vi "sheshen.vi"(3 "数组":cluster{"数值":dbl, "数值 2":dbl}[](array[cluster])) -> (1 "逻辑或":bool)   [LabVIEW 2009]
doc: "当蛇身大于等于5时判断蛇头是否和蛇身碰撞！若碰撞返回一个ture结束游戏，否则返回false游戏继续！"
uses:
  Global 3.vi
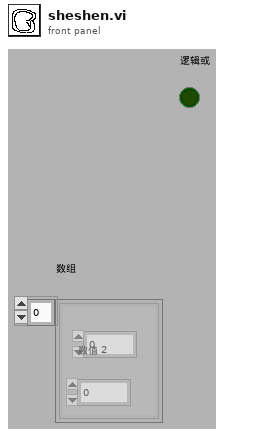
[diagram p1: front panel]
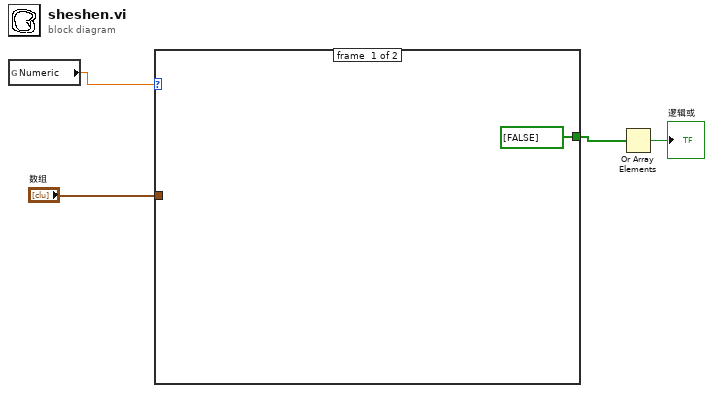
[diagram p0: block diagram]
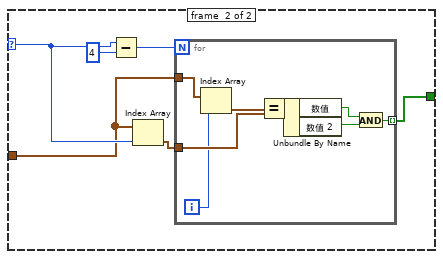
[diagram p2: hidden frame]
diagram:
  n1 = global read "Global 3.vi" "Numeric"() -> (w4:dbl)
  n2 = case shown="5, 默认" w4 {
    selector: w4 -> [_ w9]
    tunnel: "数组" -> [_ w6]
    tunnel: [bool[] [FALSE] w7] -> w2
    frame #0 {
    }
    frame #1 {
      n3 = Subtract(x=w9, y=4) -> (x-y=w10:i32)
      n4 = Index Array(array=w6, index=w9) -> (element=w8:cluster{"数值":dbl, "数值 2":dbl})
      n5 = for {
        N: w10 -> [_]
        tunnel: w6 -> [w19]
        tunnel: w8 -> [w17]
        tunnel: [w13] -> w7 mode=indexing
        i -> [w12]
        n6 = Index Array(array=w19, index=w12) -> (element=w18:cluster{"数值":dbl, "数值 2":dbl})
        n7 = Equal?(x=w18, y=w17) -> (x = y?=w16:cluster{"数值":bool, "数值 2":bool})
        n8 = Unbundle By Name(w16) -> ("数值"=w15:bool, "数值 2"=w14:bool)
        n9 = And(x=w15, y=w14) -> (x .and. y?=w13:bool)
      }
    }
  }
  n10 = Or Array Elements(Boolean array=w2) -> (logical OR=→"逻辑或":bool)
